vi "ShowBands.vi"(2 "Magnitude":T2(graph)=[{0.0, "df"=1.46484375, "Power Spectrum (V^2 rms)"=array[16384 elements]}, {0.0, "df"=1.46484375, "Power Spectrum (V^2 rms)"=array[6612 elements]}], 3 "CrsrList":T1) -> (0 "Normalized FFT":T2(graph), 1 "Cursor Data":string[][](table))   [LabVIEW 2014]
uses:
  <vilib>/Utility/miscctls.llb/LVCursorListTypeDef.ctl
  <vilib>/Analysis/baseanly.llb/Mean (DBL).vi
  <vilib>/Analysis/NI_AALBase.lvlib
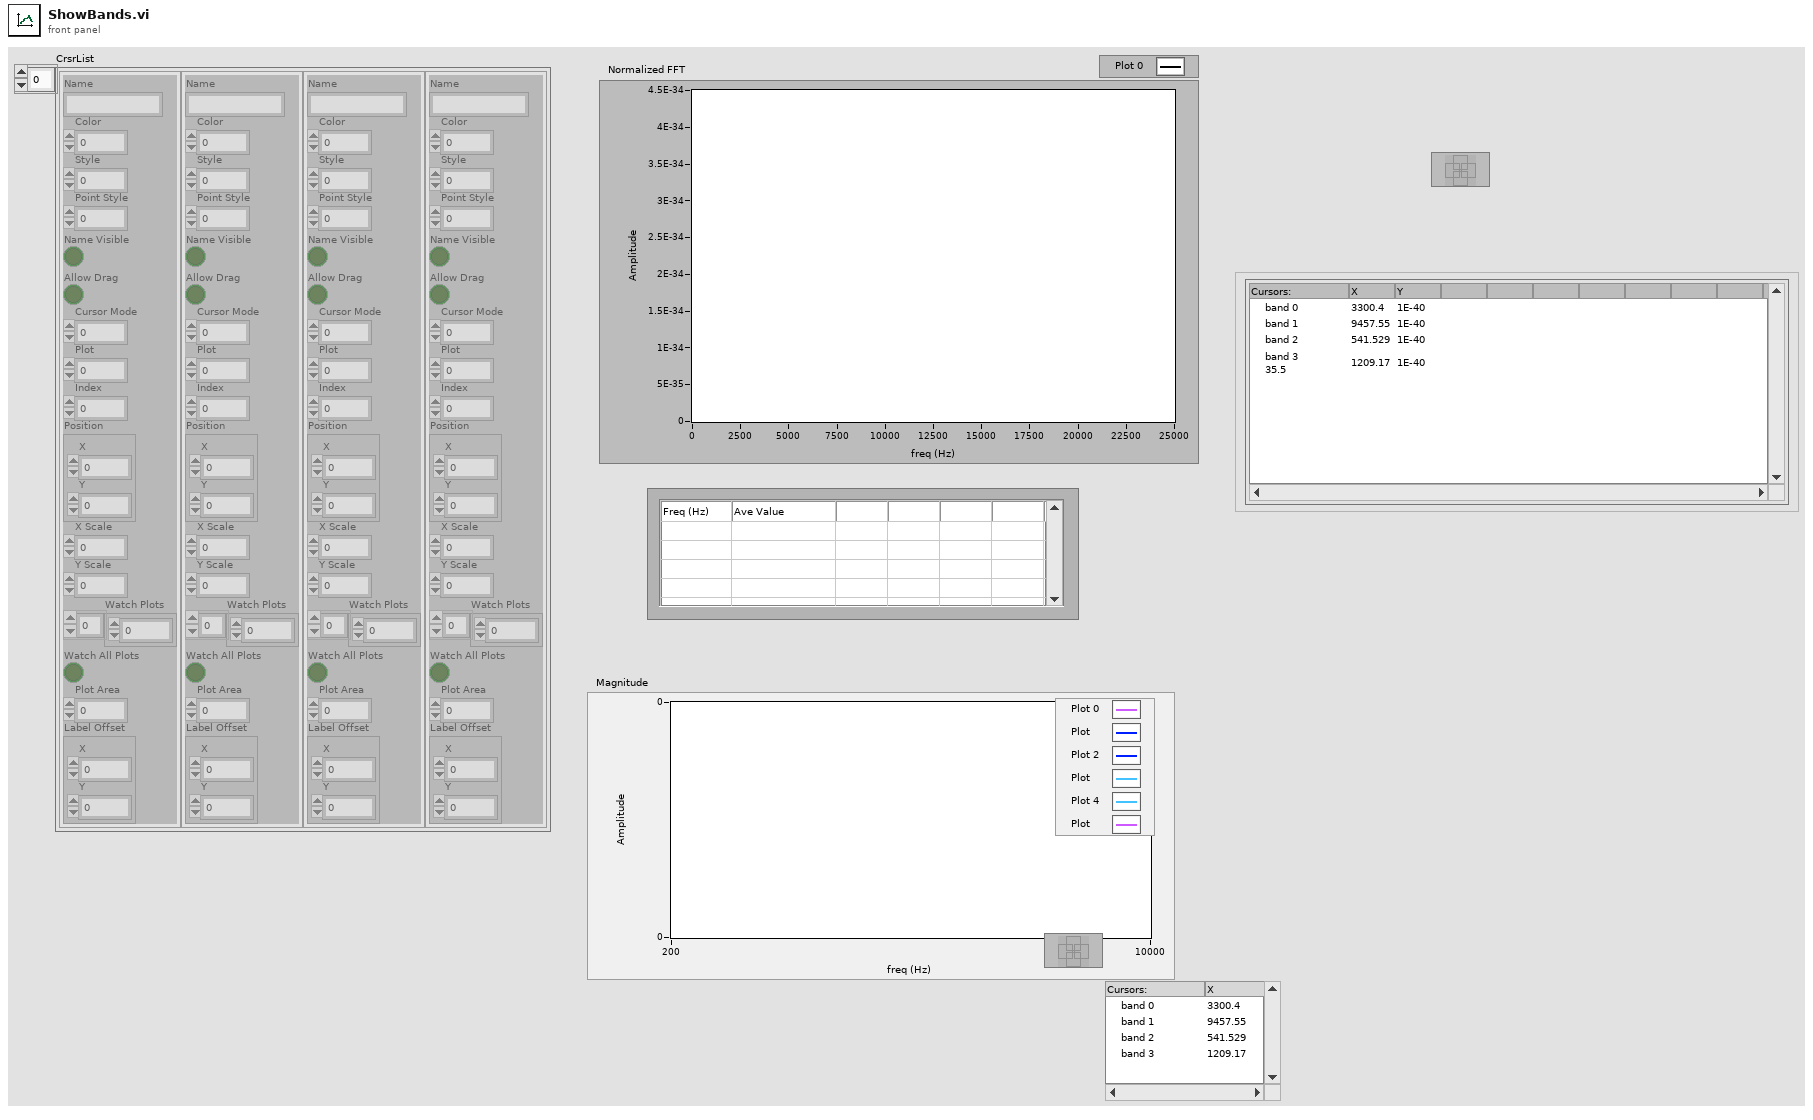
[diagram p1: front panel]
types:
  T1 = typedef "LVCursorListTypeDef.ctl" = cluster{"Name":string, "Color":u32, "Style":u8, "Point Style":u8, "Name Visible":bool, "Allow Drag":bool, "Cursor Mode":u32, "Plot":i32, "Index":i32, "Position":cluster{"X":dbl, "Y":dbl}, "X Scale":u32, "Y Scale":u32, "Watch Plots":i32[], "Watch All Plots":bool, "Plot Area":i32, "Label Offset":cluster{"X":dbl, "Y":dbl}}[]
  T2 = cluster{dbl, "df":dbl, "Power Spectrum (V^2 rms)":dbl[]}[]
  T3 = cluster{"X":dbl, cluster{"Name":string, "Color":u32, "Style":u8, "Point Style":u8, "Name Visible":bool, "Allow Drag":bool, "Cursor Mode":u32, "Plot":i32, "Index":i32, "Position":cluster{"X":dbl, "Y":dbl}, "X Scale":u32, "Y Scale":u32, "Watch Plots":i32[], "Watch All Plots":bool, "Plot Area":i32, "Label Offset":cluster{"X":dbl, "Y":dbl}}}
  T4 = cluster{"X":dbl, cluster{"Name":string, "Color":u32, "Style":u8, "Point Style":u8, "Name Visible":bool, "Allow Drag":bool, "Cursor Mode":u32, "Plot":i32, "Index":i32, "Position":cluster{"X":dbl, "Y":dbl}, "X Scale":u32, "Y Scale":u32, "Watch Plots":i32[], "Watch All Plots":bool, "Plot Area":i32, "Label Offset":cluster{"X":dbl, "Y":dbl}}}[]
  T5 = cluster{"Name":string, "Color":u32, "Style":u8, "Point Style":u8, "Name Visible":bool, "Allow Drag":bool, "Cursor Mode":u32, "Plot":i32, "Index":i32, "Position":cluster{"X":dbl, "Y":dbl}, "X Scale":u32, "Y Scale":u32, "Watch Plots":i32[], "Watch All Plots":bool, "Plot Area":i32, "Label Offset":cluster{"X":dbl, "Y":dbl}}
  T6 = cluster{dbl, "df":dbl, "Power Spectrum (V^2 rms)":dbl[]}
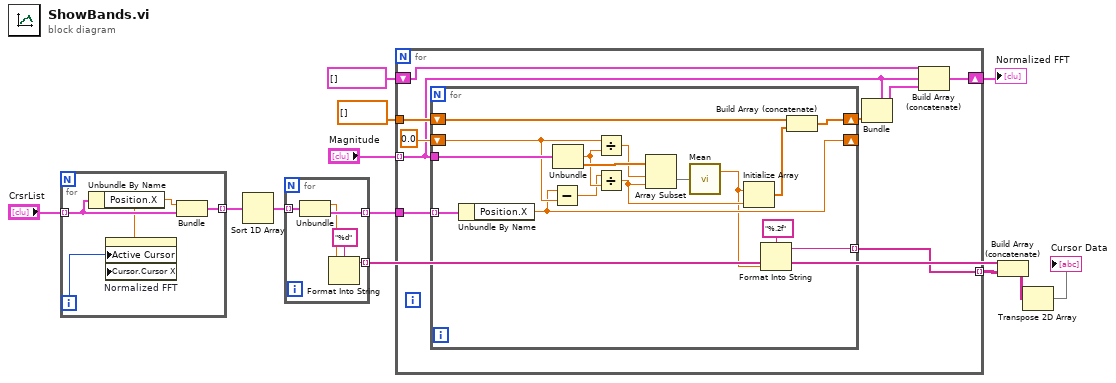
[diagram p0: block diagram]
diagram:
  n1 = for {
    tunnel: "CrsrList" -> [w16] mode=indexing
    tunnel: [w15] -> w10 mode=indexing
    i -> [w14]
    n2 = Unbundle By Name(w16) -> ("Position.X"=w13:dbl)
    n3 = property on="Normalized FFT" class="WFGraph (strict)"("Active Cursor"=w14, "Cursor.Cursor X"=w13) -> ()  [unwired: 2 in, 2 out]
    n4 = Bundle("X"=w13, w16) -> (w15:T3)  [unwired: 1 in]
  }
  n5 = Sort 1D Array(array=w10) -> (sorted array=w9:T4)
  n6 = for {
    tunnel: w9 -> [w21] mode=indexing
    tunnel: [w20] -> w7 mode=indexing
    tunnel: [w17] -> w4 mode=indexing
    n7 = Unbundle(w21) -> ("X"=w18:dbl, w20:T5)
    n8 = Format Into String(format string="%d", w18) -> (resulting string=w17:string)  [unwired: 2 in, 1 out]
  }
  n9 = for {
    tunnel: "Magnitude" -> [w25] mode=indexing
    tunnel: dbl[] [] -> [w29]
    tunnel: w7 -> [w27]
    shift-right: [w26] -> w5
    shift-left: T2 [] -> [w23]
    tunnel: [w22] -> w3 mode=indexing
    n10 = for {
      tunnel: w27 -> [w46] mode=indexing
      tunnel: w25 -> [w45]
      shift-right: [w33] -> _
      shift-left: 0.0 -> [w35]
      shift-right: [w38] -> w30
      shift-left: w29 -> [w40]
      tunnel: [w31] -> w22 mode=indexing
      n11 = Unbundle By Name(w46) -> ("Position.X"=w33:dbl)
      n12 = Subtract(x=w33, y=w35) -> (x-y=w37:dbl)
      n13 = Unbundle(w45) -> ("df"=w43:dbl, "Power Spectrum (V^2 rms)"=w44:dbl[])  [unwired: 1 out]
      n14 = Divide(x=w35, y=w43) -> (x/y=w42:dbl)
      n15 = Divide(x=w37, y=w43) -> (x/y=w41:dbl)
      n16 = Array Subset(array=w44, index=w42, length=w41) -> (w36:dbl[])
      n17 = call-poly <vilib>:"Mean.vi"("X"=w36) -> ("mean"=w32:dbl)  [unwired: 1 out]
      n18 = Initialize Array(w32, w41) -> (w39:dbl[])
      n19 = Format Into String(format string="%.2f", w32) -> (resulting string=w31:string)  [unwired: 2 in, 1 out]
      n20 = Build Array (concatenate)(w40, w39) -> (w38:dbl[])
    }
    n21 = Bundle(cluster=w25, "Power Spectrum (V^2 rms)"=w30) -> (w24:T6)  [unwired: 2 in]
    n22 = Build Array (concatenate)(w23, w25, w24) -> (w26:T2)
  }
  "Normalized FFT" <- w5
  n23 = Build Array (concatenate)(w4, w3) -> (w2:string[][])
  n24 = Transpose 2D Array(2D array=w2) -> (transposed array=→"Cursor Data":string[][])
